vi "setNSteps.vi"(7 "FWD":bool=TRUE, 8 "error in":errorcluster, 9 "setnSteps in":dbl, 10 "axis in":u8, 11 "connection ID":refnum<k5>) -> (0 "error out":errorcluster, 1 "setnSteps out":dbl, 2 "axis out":u8, 3 "connection ID":refnum<k5>)   [LabVIEW 2019]
panel:
  in  "Set Command":string="com.attocube.amc.move.setNSteps"
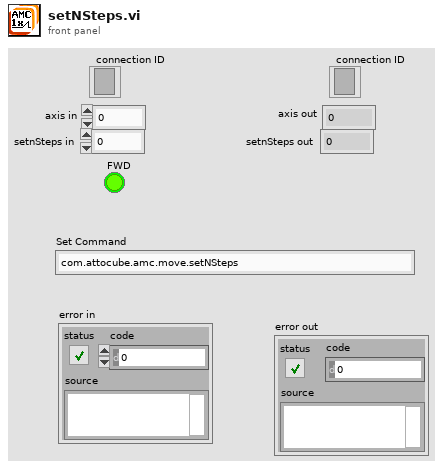
[diagram p1: front panel]
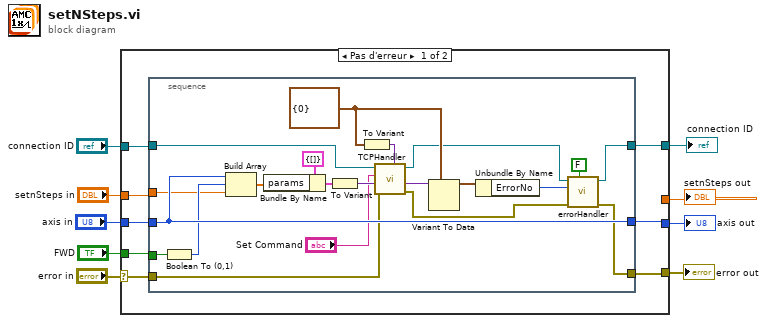
[diagram p0: block diagram]
diagram:
  n1 = case shown="Pas d'erreur" "error in" {
    selector: "error in" -> [w10 w39]
    tunnel: "axis in" -> [w15 w42]
    tunnel: [w11 w39] -> w8
    tunnel: [w12 w42] -> w7
    tunnel: "setnSteps in" -> [w17 w41]
    tunnel: [w13 w40] -> w5
    tunnel: "connection ID" -> [w14 w40]
    tunnel: "FWD" -> [w16 _]
    tunnel: [_ w41] -> w1
    frame No Error {
      n2 = stacked-sequence {
        tunnel: [w21] -> w13
        tunnel: w14 -> [w28]
        tunnel: w15 -> [w30]
        tunnel: [w30] -> w12
        tunnel: [w29] -> w11
        tunnel: w16 -> [w25]
        tunnel: w17 -> [w23]
        tunnel: w10 -> [w19]
        frame #0 {
          w26 = cluster{"ErrorNo":i64} {"ErrorNo"=0} ("input cluster")
          n3 = Boolean To (0,1)(Boolean=w25) -> (0, 1=w24:i16)
          n4 = Build Array(w30, w24, w23) -> (w34:dbl[])
          n5 = Bundle By Name(cluster=cluster{"params":i32[]} {"params"=[]} ("input cluster"), "params"=w34) -> (w35:cluster{"params":i32[]})
          n6 = To Variant(anything=w35) -> (Variant=w36:variant)
          n7 = To Variant(anything=w26) -> (Variant=w27:variant)
          n8 = call <userlib>:"TCPHandler.vi"("result Types"=w27, "error in (no error)"=w19, "params"=w36, "method"="Set Command", "connection ID"=w28) -> ("error out"=w18:errorcluster, "result"=w32:variant, "connection ID"=w22:refnum<k5>)  [unwired: 3 in, 1 out]
          n9 = Variant To Data(type=w26, Variant=w32) -> (data=w37:cluster{"ErrorNo":i64})  [unwired: 1 in, 1 out]
          n10 = Unbundle By Name(w37) -> ("ErrorNo"=w38:i64)
          n11 = call <userlib>:"errorHandler.vi"("show popup"=FALSE, "error in"=w18, "error number"=w38, "connection ID"=w22) -> ("error out"=w29:errorcluster, "connection ID"=w21:refnum<k5>)  [unwired: 6 in]
        }
      }
    }
    frame Error {
    }
  }
  "error out" <- w8
  "axis out" <- w7
  "setnSteps out" <- w1
  "connection ID" <- w5
